vi "TestOpenCycle.vi"() -> ()   [LabVIEW 2023]
uses:
  S7Plc.ctl
  D:/Projects/S7View/S7Lib/bin/Debug/S7.Net.dll
  S7Lib/bin/Debug/S7.Net.dll
panel:
  out "S7PLC 2":T1={"ip"="192.168.10.10", "type"=40, "rack"=0, "slot"=0, "status"=FALSE, "link"=FALSE, "msg"="", "plc"=refnum} caption="S7PLC" {"type" items=["S7200"=0, "Logo0BA8"=1, "S7200Smart"=2, "S7300"=10, "S7400"=20, "S71200"=30, "S71500"=40]}
  in  "等待时间（毫秒）":u32
  in  "布尔":bool
  out "S7PLC":T1={"ip"="192.168.10.10", "type"=40, "rack"=0, "slot"=0, "status"=FALSE, "link"=FALSE, "msg"="", "plc"=refnum} {"type" items=["S7200"=0, "Logo0BA8"=1, "S7200Smart"=2, "S7300"=10, "S7400"=20, "S71200"=30, "S71500"=40]}
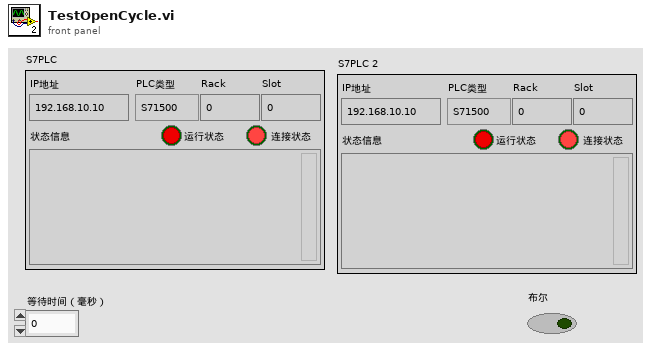
[diagram p1: front panel]
types:
  T1 = typedef "S7Plc.ctl" = cluster{"ip":string, "type":i16, "rack":i16, "slot":i16, "status":bool, "link":bool, "msg":string, "plc":refnum<k24>}
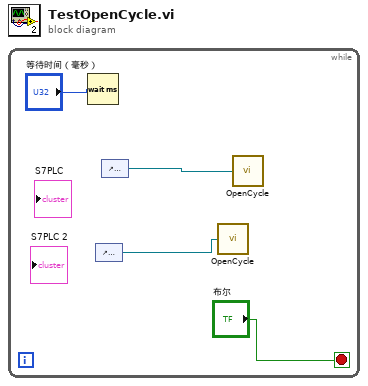
[diagram p0: block diagram]
diagram:
  n1 = while {
    stop <- "布尔" stop-if-true
    n2 = Wait (ms)(milliseconds to wait="等待时间（毫秒）") -> ()  [unwired: 1 out]
    n3 = control-ref of="S7PLC 2"() -> (w1:refnum<vi>)
    n4 = control-ref of="S7PLC"() -> (w2:refnum<vi>)
    n5 = call "OpenCycle.vi"("PLC"=w1) -> ()
    n6 = call "OpenCycle.vi"("PLC"=w2) -> ()
  }
